vi "Is Running.vi"(0 "eye scan in":refnum<class "niHighSpeedSerial Eye Scan v1 Host.lvclass">, 11 "error in":errorcluster) -> (4 "eye scan out":refnum<class "niHighSpeedSerial Eye Scan v1 Host.lvclass">, 6 "is running?":bool, 15 "error out":errorcluster)   [LabVIEW 2014, in "niHighSpeedSerial Eye Scan v1 Host.lvclass"]
doc: "Returns true if the Eye Scan session is currently in the Running state.\n\n<B>Input Parameters</B>\n\n<B>eye scan in</B> Takes in a reference to your session from the previous VI.\n\n<B>error in</B> describes error conditions that occur before this node runs. This input provides standard 'error in' functionality.\n\n<B>Output Parameters</B>\n\n<B>eye scan out</B> passes a reference to your session to the next VI.\n\n<B>is running?</B> True if the session is currently in the running state.\n\n<B>error out</B> contains error information. This output provides standard 'error out' functionality."
uses:
  <instrlib>/niHighSpeedSerial/Eye Scan/v1/Host/Eye Scan/niHighSpeedSerial Eye Scan v1 Host.lvclass
  <instrlib>/niHighSpeedSerial/Eye Scan/v1/Host/Eye Scan/niHighSpeedSerial Eye Scan v1 Host.lvclass/niHighSpeedSerial Eye Scan v1 Host.ctl
  <instrlib>/niHighSpeedSerial/Eye Scan/v1/Host/Eye Scan/Private/Measure State.ctl
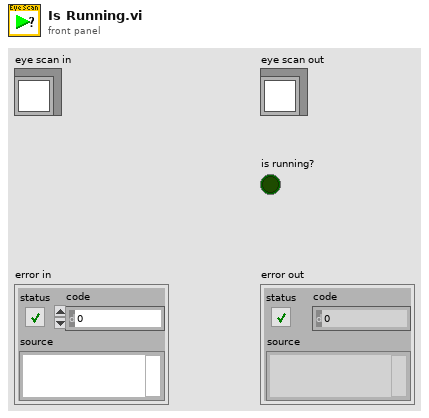
[diagram p1: front panel]
types:
  T1 = typedef "niHighSpeedSerial Eye Scan v1 Host.lvclass/Measure State.ctl" = enum16{"Uninitialized", "Initialized", "Ready", "Measuring", "Finished", "Aborted"}
  T2 = typedef "niHighSpeedSerial Eye Scan v1 Host.lvclass/Private Data.ctl" = cluster{"instruction target":refnum<class "niInstr Instruction Target v1 Host.lvclass">, "channels":T3[], "measure state":T1, "rx output divider":T4, "equalization mode":T5, "rx data width":T6, "BER floor":dbl, "number of points completed":i32, "rx output divider configured?":bool, "equalization mode configured?":bool, "rx data width configured?":bool}
  T3 = typedef "niHighSpeedSerial Eye Scan v1 Host.lvclass/Channel Data.ctl" = cluster{"instance":u8, "channel":refnum<class "niHighSpeedSerial Eye Scan Single Point v1 Host.lvclass">, "point iterator":refnum<class "niHighSpeedSerial Eye Scan Point Iterator v1 Host.lvclass">}
  T4 = typedef "niHighSpeedSerial Eye Scan Common v1 Host.lvlib/RX Output Divider.ctl" = enum16{"1", "2", "4", "8", "16"}
  T5 = typedef "niHighSpeedSerial Eye Scan Common v1 Host.lvlib/Equalization Mode.ctl" = enum16{"DFE", "LPM"}
  T6 = typedef "niHighSpeedSerial Eye Scan Common v1 Host.lvlib/Data Width.ctl" = enum16{"16 Bit", "20 Bit", "32 Bit", "40 Bit"}
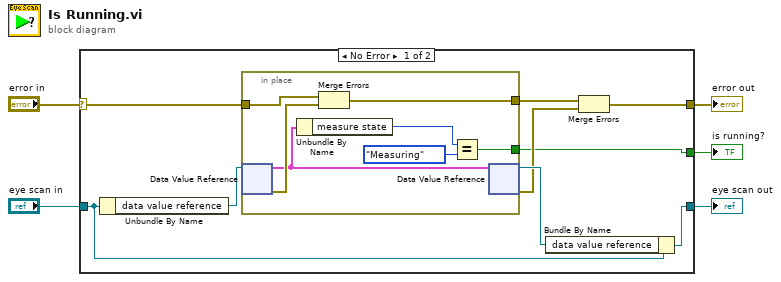
[diagram p0: block diagram]
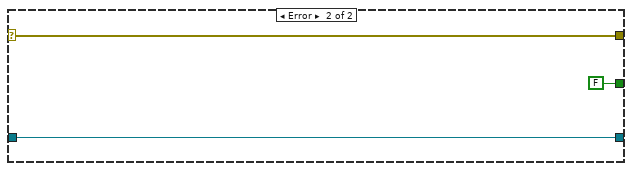
[diagram p2: hidden frame]
diagram:
  n1 = case shown="No Error" "error in" {
    selector: "error in" -> [w10 w24]
    tunnel: [w7 w24] -> w4
    tunnel: [w11 w23] -> w3
    tunnel: "eye scan in" -> [w13 w23]
    tunnel: [w6 FALSE ("is running?")] -> w1
    frame No Error {
      n2 = Unbundle By Name(w13) -> ("data value reference"=w14:refnum<data-value>)
      n3 = in-place {
        in-place-border: w10 -> [w21]
        in-place-border: [w19] -> w8
        in-place-border: [w16] -> w6
        n4 = in-place-dvr #1(w14) -> (w15:T2, w20:errorcluster)
        n5 = Unbundle By Name(w15) -> ("measure state"=w18:T1)
        n6 = Merge Errors(w21, w20) -> (w19:errorcluster)
        n7 = Equal?(x=w18, y=Measure_State."Measuring") -> (x = y?=w16:bool)
        n8 = in-place-dvr #1(w15) -> (w12:refnum<data-value>, w9:errorcluster)
      }
      n9 = Bundle By Name(cluster=w13, "data value reference"=w12) -> (w11:refnum<class "niHighSpeedSerial Eye Scan v1 Host.lvclass">)
      n10 = Merge Errors(w8, w9) -> (w7:errorcluster)
    }
    frame Error {
    }
  }
  "error out" <- w4
  "eye scan out" <- w3
  "is running?" <- w1
